vi "public_device_unoccupy_choose_step.vi"(8 "error In":errorcluster, 9 "JSON string":string, 10 "Step order":string, 11 "process_ID":string) -> (0 "error IO":errorcluster)   [LabVIEW 2020]
uses:
  status/public_device_list.vi
  status/status of robot.vi
  status/status of pump.vi
  status/status of relay.vi
  status/emergency stop.vi
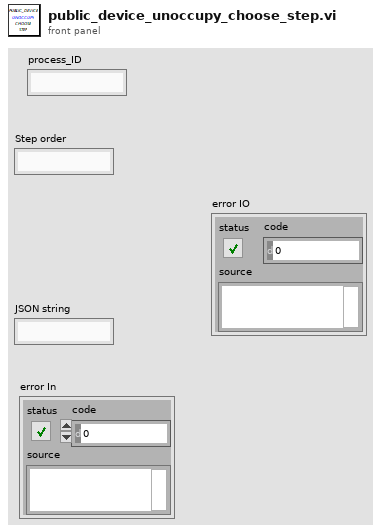
[diagram p1: front panel]
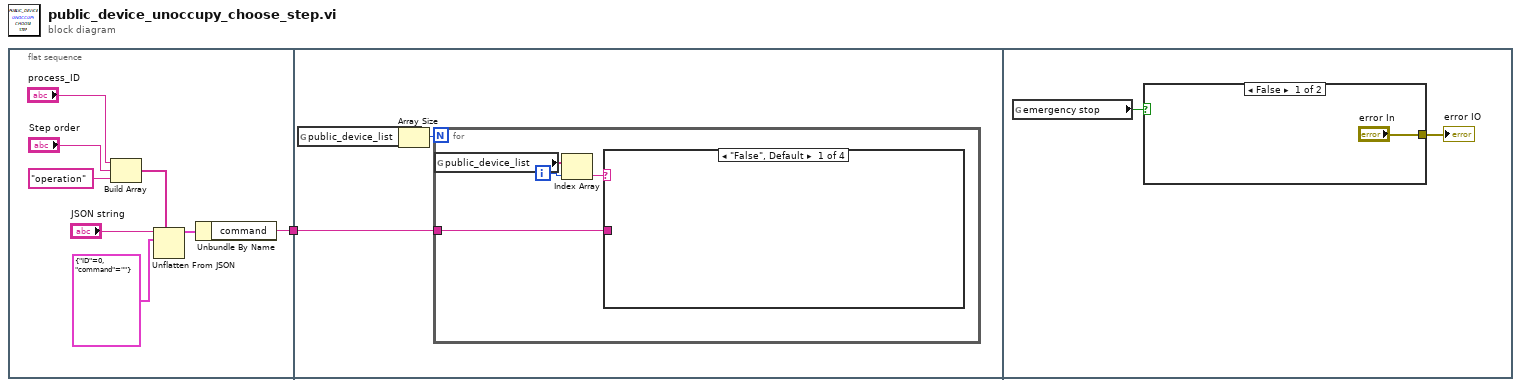
[diagram p0: block diagram]
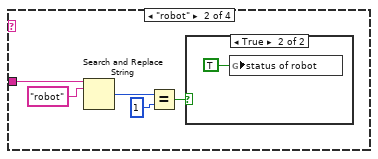
[diagram p2: hidden frame]
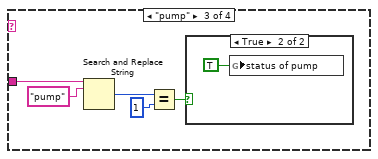
[diagram p4: hidden frame]
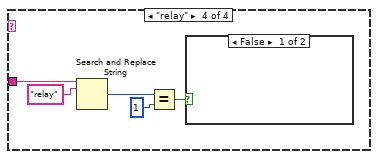
[diagram p6: hidden frame]
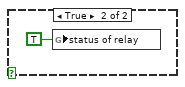
[diagram p7: hidden frame]
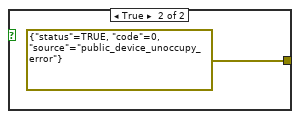
[diagram p8: hidden frame]
diagram:
  n1 = flat-sequence {
    tunnel: [w4] -> w1
    tunnel: w1 -> [w10]
    frame #0 {
      n2 = Build Array("process_ID", "Step order", "operation" ("string")) -> (w7:string[])
      n3 = Unflatten From JSON(path=w7, JSON string="JSON string", type and defaults=cluster{"ID":u8, "command":string} {"ID"=0, "command"=""} ("参数")) -> (value=w5:cluster{"ID":u8, "command":string})  [unwired: 4 in, 1 out]
      n4 = Unbundle By Name(w5) -> ("command"=w4:string)
    }
    frame #1 {
      n5 = global read "public_device_list.vi" "public_device_list"() -> (w12:string[])
      n6 = Array Size(array=w12) -> (size(s)=w11:i32)
      n7 = for {
        N: w11 -> [_]
        tunnel: w10 -> [w13]
        i -> [w15]
        n8 = global read "public_device_list.vi" "public_device_list"() -> (w16:string[])
        n9 = Index Array(array=w16, index=w15) -> (element=w14:string)
        n10 = case shown="\"False\", Default" w14 {
          tunnel: w13 -> [_ w17 w23 w29]
          frame "False", Default {
          }
          frame "robot" {
            n11 = Search and Replace String(input string=w17, search string="robot") -> (number of replacements=w21:i32)  [unwired: 6 in, 3 out]
            n12 = Equal?(x=w21, y=1) -> (x = y?=w18:bool)
            n13 = case shown="True" w18 {
              frame False {
              }
              frame True {
                n14 = global write "status of robot.vi" "status of robot"(TRUE ("status of robot")) -> ()
              }
            }
          }
          frame "pump" {
            n15 = Search and Replace String(input string=w23, search string="pump") -> (number of replacements=w27:i32)  [unwired: 6 in, 3 out]
            n16 = Equal?(x=w27, y=1) -> (x = y?=w24:bool)
            n17 = case shown="True" w24 {
              frame False {
              }
              frame True {
                n18 = global write "status of pump.vi" "status of pump"(TRUE ("status of pump")) -> ()
              }
            }
          }
          frame "relay" {
            n19 = Search and Replace String(input string=w29, search string="relay") -> (number of replacements=w33:i32)  [unwired: 6 in, 3 out]
            n20 = Equal?(x=w33, y=1) -> (x = y?=w30:bool)
            n21 = case shown="False" w30 {
              frame False {
              }
              frame True {
                n22 = global write "status of relay.vi" "status of relay"(TRUE ("status of relay")) -> ()
              }
            }
          }
        }
      }
    }
    frame #2 {
      n23 = global read "emergency stop.vi" "emergency stop"() -> (w35:bool)
      n24 = case shown="False" w35 {
        tunnel: ["error In" errorcluster {"status"=TRUE, "code"=0, "source"="public_device_unoccupy_error"} ("error IO")] -> w36
        frame False {
        }
        frame True {
        }
      }
      "error IO" <- w36
    }
  }
